vi "Reserve UART.vi"(7 "UART Pins":T1={"TX GPIO"=-1, "RX GPIO"=-1}, 8 "error in (no error)":errorcluster, 9 "Purpose":string, 10 "UART #":T3=-1, 11 "Session in":refnum<class "Session.lvclass">) -> (0 "error out":errorcluster, 2 "UART":refnum<class "UART.lvclass">, 3 "Session out":refnum<class "Session.lvclass">)   [LabVIEW 2020, in "CTI.lvlib" / "Session.lvclass"]
uses:
  Session.lvclass
  UART Number.ctl
  UART/UART.lvclass
  C:/dev/cti/cti-drivers-lv-visa/CTI/Resource/Resource.lvclass
  UART Pins.ctl
  GPIO Number.ctl
  Resource/Resource.lvclass/Resource.ctl
  Session.lvclass/Session.ctl
  dcef0d26-6755-4235-b060-6b0e00c3d74f.vi
  dcef0d26-6755-4235-b060-6b0e00c3d74f.vi/685f7f19-b444-4620-8f66-e6e2ddd64bb8.vi
  Generate Error.vi
  GPIO/GPIO.lvclass
  Resource/Resource.lvclass
  CTI.lvlib
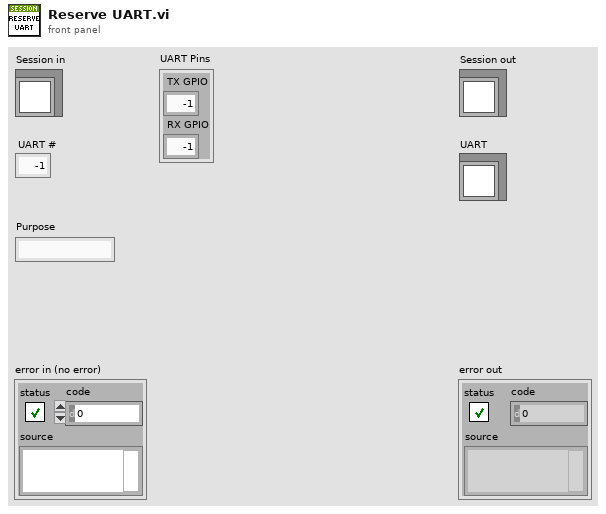
[diagram p1: front panel]
types:
  T1 = typedef "CTI.lvlib/UART Pins.ctl" = cluster{"TX GPIO":T2, "RX GPIO":T2}
  T2 = typedef "CTI.lvlib/GPIO Number.ctl" = i8
  T3 = typedef "CTI.lvlib/UART Number.ctl" = i8
  T4 = typedef "CTI.lvlib/Session.lvclass/Resources.ctl" = cluster{"GPIO":map{T2, refnum<class "GPIO.lvclass">}, "AI":map{T5, refnum<class "AI.lvclass">}, "PWM":map{T2, refnum<class "PWM.lvclass">}, "UART":map{T3, refnum<class "UART.lvclass">}, "I2C":map{T6, refnum<class "I2C.lvclass">}, "SPI":map{T7, refnum<class "SPI.lvclass">}, "CS":map{T2, refnum<class "SPI CS.lvclass">}}
  T5 = typedef "CTI.lvlib/ADC Number.ctl" = i8
  T6 = typedef "CTI.lvlib/I2C Number.ctl" = i8
  T7 = typedef "CTI.lvlib/SPI Number.ctl" = i8
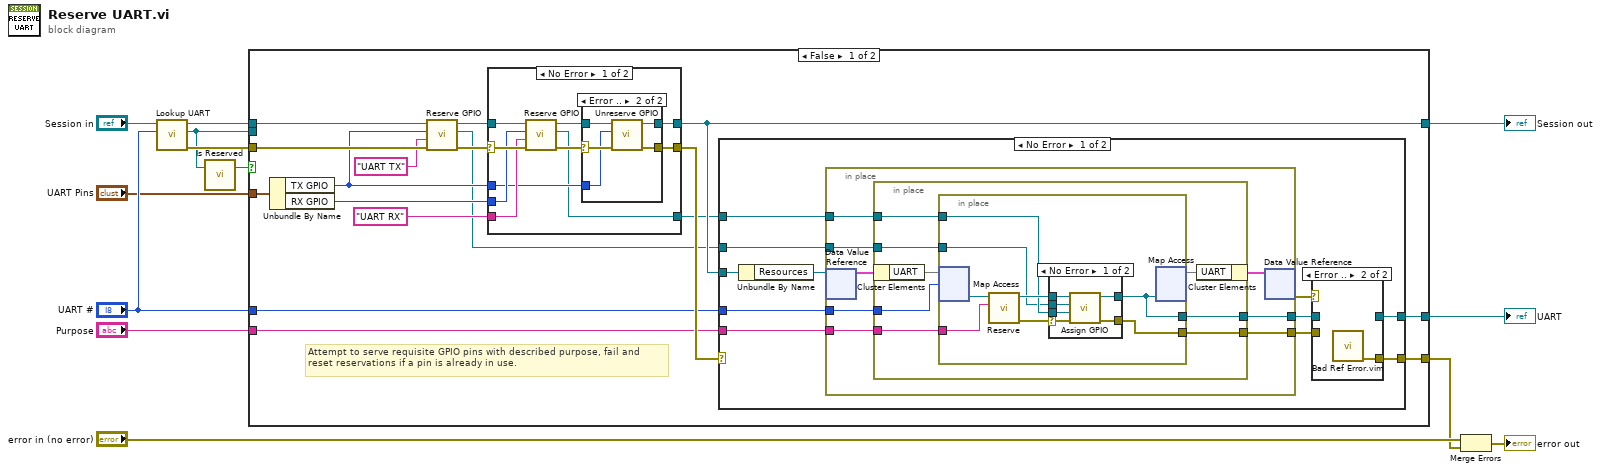
[diagram p0: block diagram]
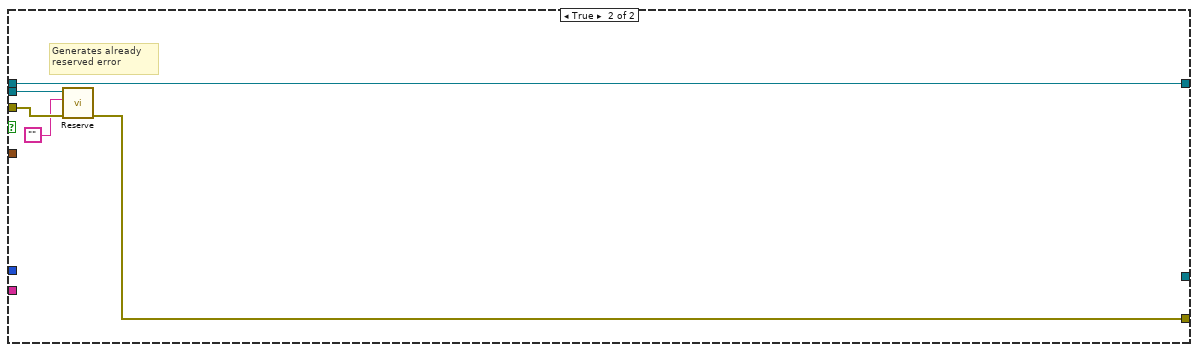
[diagram p7: hidden frame]
diagram:
  n1 = call "Lookup UART.vi"("UART #"="UART #", "Session in"="Session in") -> ("error out"=w13:errorcluster, "UART"=w1:refnum<class "UART.lvclass">, "Session out"=w6:refnum<class "Session.lvclass">)  [unwired: 7 in]
  n2 = call "Is Reserved.vi"("Resource in"=w1) -> ("Reserved"=w2:bool)  [unwired: 6 in]
  n3 = case shown="False" w2 {
    tunnel: w13 -> [w28 w100]
    tunnel: "Purpose" -> [w27 _]
    tunnel: [w26 _] -> w10
    tunnel: [w25 w98] -> w7
    tunnel: w6 -> [w24 w99]
    tunnel: "UART #" -> [w23 _]
    tunnel: "UART Pins" -> [w21 _]
    tunnel: [w19 w99] -> w3
    tunnel: w1 -> [_ w101]
    frame False {
      # "Attempt to serve requisite GPIO pins with described purpose, fail and reset reservations if a pin is already in use."
      n4 = Unbundle By Name(w21) -> ("TX GPIO"=w16:T2, "RX GPIO"=w18:T2)
      n5 = call "Reserve GPIO.vi"("error in (no error)"=w28, "Purpose"="UART TX", "GPIO #"=w16, "Session in"=w24) -> ("error out"=w29:errorcluster, "GPIO"=w14:refnum<class "GPIO.lvclass">, "Session out"=w20:refnum<class "Session.lvclass">)  [unwired: 5 in]
      n6 = case shown="No Error" w29 {
        selector: w29 -> [w40 w48]
        tunnel: [w33 w48] -> w30
        tunnel: w20 -> [w39 w49]
        tunnel: [w34 w49] -> w19
        tunnel: w18 -> [w38 _]
        tunnel: "UART RX" ("Purpose") -> [w37 _]
        tunnel: w16 -> [w32 _]
        tunnel: [w31 _] -> w15
        frame No Error {
          n7 = call "Reserve GPIO.vi"("error in (no error)"=w40, "Purpose"=w37, "GPIO #"=w38, "Session in"=w39) -> ("error out"=w36:errorcluster, "GPIO"=w31:refnum<class "GPIO.lvclass">, "Session out"=w35:refnum<class "Session.lvclass">)  [unwired: 5 in]
          n8 = case shown="Error .." w36 {
            selector: w36 -> [w41 w46]
            tunnel: w35 -> [w42 w47]
            tunnel: [w42 w43] -> w34
            tunnel: [w41 w44] -> w33
            tunnel: w32 -> [_ w45]
            frame No Error {
            }
            frame Error {
              n9 = call "Unreserve GPIO.vi"("error in (no error)"=w46, "GPIO #"=w45, "Session in"=w47) -> ("error out"=w44:errorcluster, "Session out"=w43:refnum<class "Session.lvclass">)  [unwired: 7 in]
            }
          }
        }
        frame Error {
        }
      }
      n10 = case shown="No Error" w30 {
        selector: w30 -> [_ w96]
        tunnel: w27 -> [w59 _]
        tunnel: [w55 _] -> w26
        tunnel: [w54 w96] -> w25
        tunnel: w23 -> [w53 _]
        tunnel: w19 -> [w52 _]
        tunnel: w15 -> [w51 _]
        tunnel: w14 -> [w50 _]
        frame No Error {
          n11 = Unbundle By Name(w52) -> ("Resources"=w60:refnum<data-value>)
          n12 = in-place {
            in-place-border: w53 -> [w71]
            in-place-border: w59 -> [w70]
            in-place-border: [w69] -> w58
            in-place-border: [w66] -> w56
            in-place-border: w51 -> [w65]
            in-place-border: w50 -> [w64]
            n13 = in-place-dvr #1(w60) -> (w67:T4)  [unwired: 1 out]
            n14 = in-place {
              in-place-border: w71 -> [w78]
              in-place-border: w70 -> [w77]
              in-place-border: [w76] -> w69
              in-place-border: [w74] -> w66
              in-place-border: w65 -> [w73]
              in-place-border: w64 -> [w72]
              n15 = in-place-cluster #2(w67) -> ("UART"=w79:map{T3, refnum<class "UART.lvclass">})
              n16 = in-place {
                in-place-border: w77 -> [w86]
                in-place-border: [w80] -> w76
                in-place-border: [w84] -> w74
                in-place-border: w73 -> [w82]
                in-place-border: w72 -> [w81]
                n17 = in-place-map #3(w79, w78) -> (w87:refnum<class "UART.lvclass">)  [unwired: 1 in, 1 out]
                n18 = call "Reserve.vi"("Purpose"=w86, "Resource in"=w87) -> ("error out"=w83:errorcluster, "Resource out"=w85:refnum<class "UART.lvclass">)  [unwired: 8 in]
                n19 = case shown="No Error" w83 {
                  selector: w83 -> [w91 w95]
                  tunnel: w85 -> [w93 w94]
                  tunnel: [w92 w94] -> w84
                  tunnel: w82 -> [w90 _]
                  tunnel: w81 -> [w89 _]
                  tunnel: [w88 w95] -> w80
                  frame No Error {
                    n20 = call "Assign GPIO.vi"("error in (no error)"=w91, "RX"=w90, "TX"=w89, "UART in"=w93) -> ("error out"=w88:errorcluster, "UART out"=w92:refnum<class "UART.lvclass">)  [unwired: 6 in]
                  }
                  frame Error {
                  }
                }
                n21 = in-place-map #3(w84) -> (w75:map{T3, refnum<class "UART.lvclass">})  [unwired: 1 in, 2 out]
              }
              n22 = in-place-cluster #2("UART"=w75) -> (w68:T4)
            }
            n23 = in-place-dvr #1(w68) -> (w57:errorcluster)  [unwired: 1 out]
          }
          n24 = case shown="Error .." w57 {
            tunnel: w58 -> [w62 _]
            tunnel: [w62 w63] -> w54
            tunnel: w56 -> [w61 _]
            tunnel: [w61 _] -> w55
            frame No Error {
            }
            frame Error {
              n25 = call "Bad Ref Error.vim"() -> ("error out"=w63:errorcluster)  [unwired: 10 in, 1 out]
            }
          }
        }
        frame Error {
          # "Error generated reserving GPIO Pin(s) or looking up I2C #"
        }
      }
    }
    frame True {
      # "Generates already reserved error"
      n26 = call "Reserve.vi"("error in (no error)"=w100, "Purpose"="", "Resource in"=w101) -> ("error out"=w98:errorcluster)  [unwired: 7 in, 1 out]
    }
  }
  "Session out" <- w3
  "UART" <- w10
  n27 = Merge Errors("error in (no error)", w7) -> (→"error out":errorcluster)
